vi "Simple DC Motor Control_test - Copy.vi"() -> ()   [LabVIEW 2013]
panel:
  in  "Tab Control":enum32{"DC Motor"}(tab)
  in  "STOP":bool
  in  "Direction":u16(ring) items=["Clockwise", "Counter-Clockwise"]
  in  "STOP":bool
  # "DC Motor Controller"
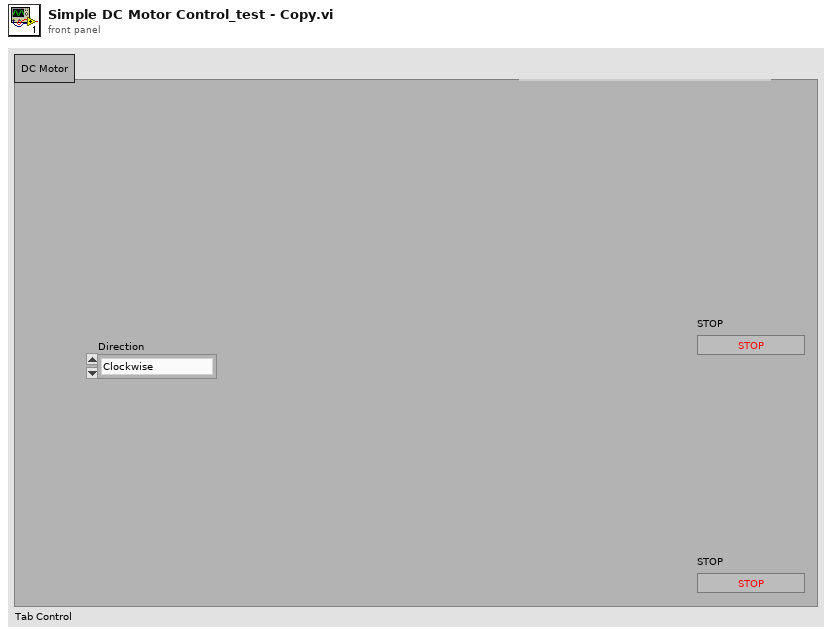
[diagram p1: front panel]
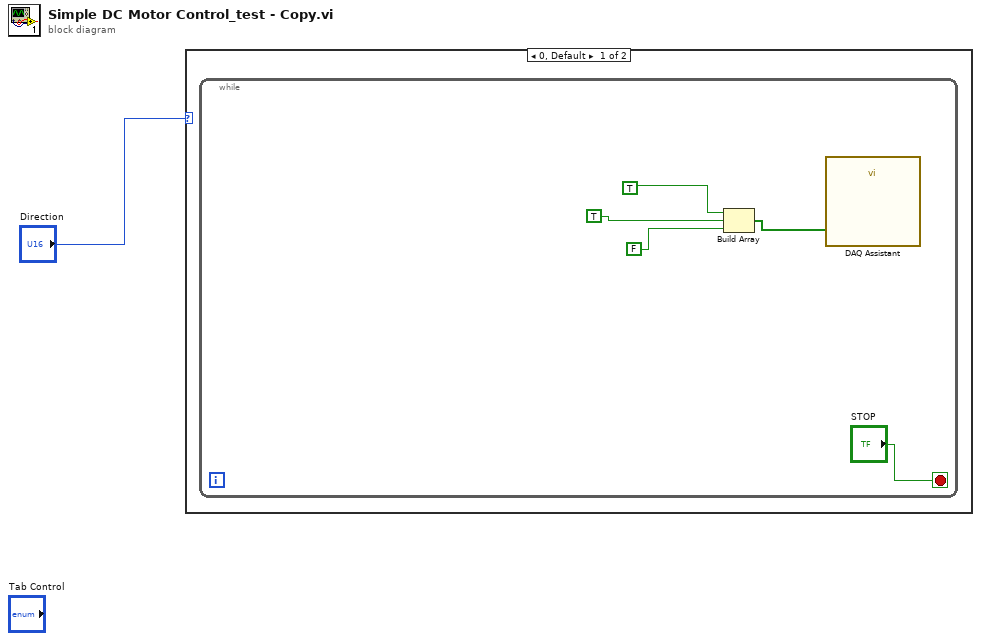
[diagram p0: block diagram]
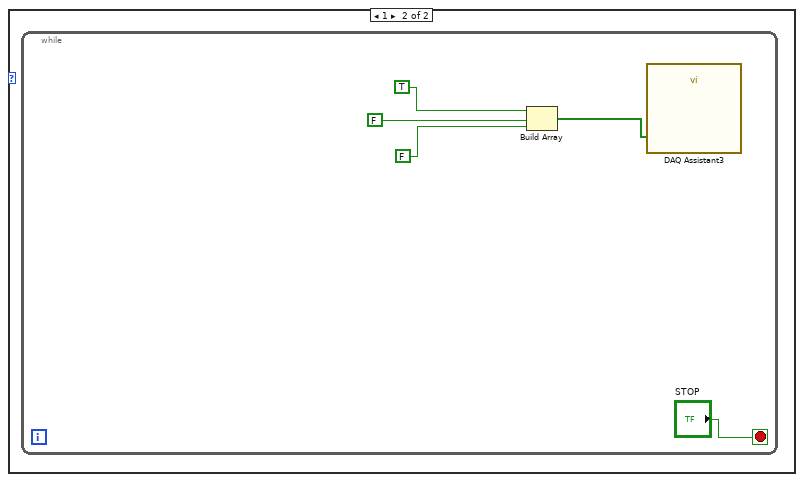
[diagram p2: hidden frame]
diagram:
  n1 = case shown="0, Default" "Direction" {
    frame 0, Default {
      n2 = while {
        stop <- "STOP" stop-if-true
        n3 = Build Array(TRUE ("Boolean"), TRUE, FALSE) -> (w6:bool[])
        n4 = call "DAQ Assistant"("data"=w6) -> ()  [unwired: 17 in, 2 out]
      }
    }
    frame 1 {
      n5 = while {
        stop <- "STOP" stop-if-true
        n6 = Build Array(TRUE, FALSE, FALSE) -> (w8:bool[])
        n7 = call "DAQ Assistant3"("data"=w8) -> ()  [unwired: 17 in, 2 out]
      }
    }
  }
